vi "tcs shm ack Command stop LV.vi"(8 "error in (no error)":errorcluster, 11 "ackcmd_Ctl":T1) -> (0 "error out":errorcluster, 2 "function return":i32, 3 "ackcmd_Ctl out":T1)   [LabVIEW 2016, in "SALLV_tcs.lvlib"]
doc: "int tcs_shm_ackCommand_stopLV(tcs_ackcmdLV *ackcmd_Ctl);"
uses:
  SALLV_tcs.lvlib
  SALLV_tcs.so
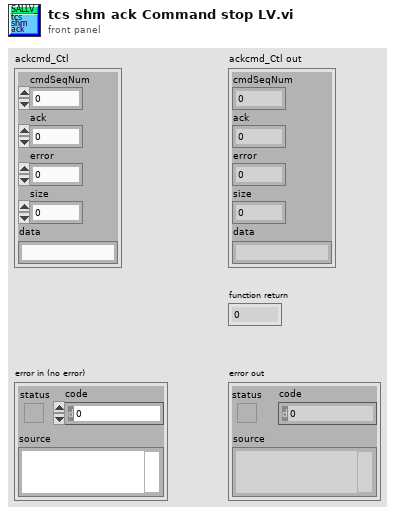
[diagram p1: front panel]
types:
  T1 = cluster{"cmdSeqNum":i32, "ack":i32, "error":i32, "size":i32, "data":string}
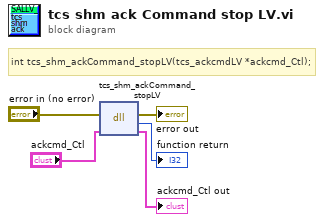
[diagram p0: block diagram]
diagram:
  # "int tcs_shm_ackCommand_stopLV(tcs_ackcmdLV *ackcmd_Ctl);"
  n1 = dll-call lib="home/plotz/SALLV_tcs/SALLV_tcs.*" fn="tcs_shm_ackCommand_stopLV"(error in="error in (no error)", "ackcmd_Ctl"="ackcmd_Ctl") -> (error out=→"error out":errorcluster, →"function return":i32, "ackcmd_Ctl"=→"ackcmd_Ctl out":T1)  [unwired: 2 in, 1 out]
